vi "Get Start Tag.vi"(8 "error in (no error)":errorcluster, 10 "Name":string, 11 "Element in":refnum<class "Element.lvclass">) -> (0 "error out":errorcluster, 2 "Start Tag":string, 3 "Element out":refnum<class "Element.lvclass">)   [LabVIEW 2026, in "VILab.lvlib" / "Element.lvclass"]
uses:
  Element.lvclass
  Attribute/Attribute.lvclass
  VILab.lvlib
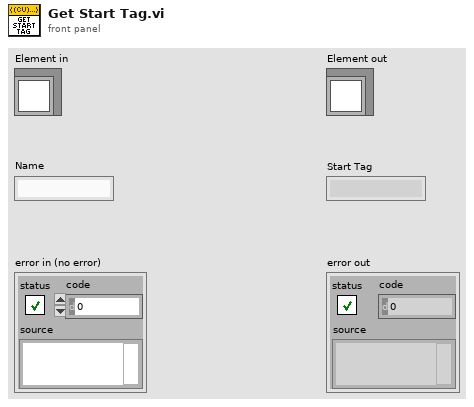
[diagram p1: front panel]
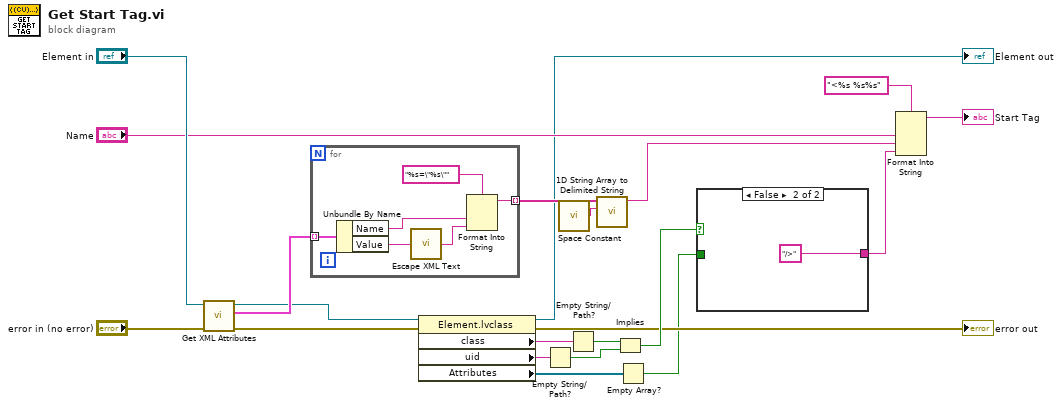
[diagram p0: block diagram]
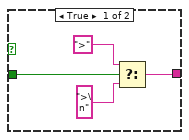
[diagram p2: hidden frame]
diagram:
  n1 = call-dynamic "Get XML Attributes.vi"("error in (no error)"="error in (no error)", "Element in"="Element in") -> ("error out"=w7:errorcluster, "XML Attributes"=w19:cluster{"Name":string, "Value":string}[], "Element out"=w6:refnum<class "Element.lvclass">)  [unwired: 7 in]
  n2 = for {
    tunnel: w19 -> [w27] mode=indexing
    tunnel: [w22] -> w15 mode=indexing
    n3 = Unbundle By Name(w27) -> ("Name"=w23:string, "Value"=w26:string)
    n4 = call "Escape XML Text.vi"("String"=w26) -> ("Escaped"=w24:string)
    n5 = Format Into String(format string="%s=\"%s\"", w23, w24) -> (resulting string=w22:string)  [unwired: 2 in, 1 out]
  }
  n6 = property class="Element.lvclass"(reference=w6, error in=w7) -> (reference out=→"Element out":refnum<class "Element.lvclass">, error out=→"error out":errorcluster, "class"=w12:string, "uid"=w11:string, "Attributes"=w3:refnum<class "Attribute.lvclass">[])
  n7 = Empty String/Path?(string/path=w11) -> (empty?=w9:bool)
  n8 = call <vilib>:"Space Constant.vi"() -> ("String"=w17:string)
  n9 = Empty String/Path?(string/path=w12) -> (empty?=w10:bool)
  n10 = call <vilib>:"1D String Array to Delimited String.vi"("delimiter"=w17, "string array"=w15) -> ("delimited string"=w16:string)  [unwired: 9 in]
  n11 = Implies(1:w9, 2:w10) -> (0:w8:bool)
  n12 = Empty Array?(array=w3) -> (empty?=w1:bool)
  n13 = case shown="False" w8 {
    tunnel: [w29 "/>"] -> w2
    tunnel: w1 -> [w28 _]
    frame True {
      n14 = Select(t=">", s=w28, f=">\n") -> (s? t:f=w29:string)
    }
    frame False {
    }
  }
  n15 = Format Into String(format string="<%s %s%s", "Name", w16, w2) -> (resulting string=→"Start Tag":string)  [unwired: 2 in, 1 out]
